vi "Write Service Name.vi"(10 "Service Name":string, 11 "Assert Service in":refnum<class "Assert Service.lvclass">) -> (3 "Assert Service out":refnum<class "Assert Service.lvclass">)   [LabVIEW 2016, in "Assert API Components.lvlib" / "Assert Service.lvlib" / "Assert Service.lvclass"]
uses:
  Assert Service.lvclass
  Assert Service.lvclass/Assert Service.ctl
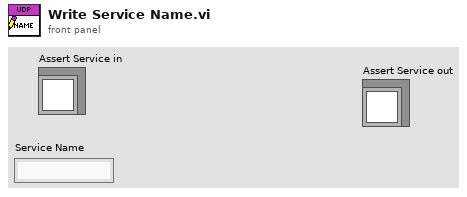
[diagram p1: front panel]
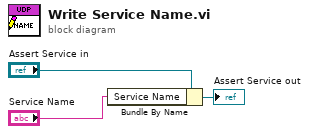
[diagram p0: block diagram]
diagram:
  n1 = Bundle By Name(cluster="Assert Service in", "Service Name"="Service Name") -> (→"Assert Service out":refnum<class "Assert Service.lvclass">)
